vi "Create Output Channels.vi"(8 "error in (no error)":errorcluster, 11 "DAQmx Lockin Digitizer Driver in":refnum<class "DAQmx Synthesizer.lvclass">) -> (0 "error out":errorcluster, 3 "DAQmx Lockin Digitizer Driver out":refnum<class "DAQmx Synthesizer.lvclass">)   [LabVIEW 2021, in "DAQmx Synthesizer.lvclass"]
uses:
  DAQmx Synthesizer.lvclass
  C:/GitHub/NHMFL_Core/Libraries/Instruments/Pulse Driver/Lockin Digitizer Driver/Lockin Digitizer Driver.lvclass
  C:/GitHub/NHMFL_Core/Libraries/NI-DAQ/DAQmx Digitizer/DAQmx Digitizer.lvclass
  C:/GitHub/NHMFL_Core/Libraries/Instruments/Pulse Driver/Pulse Driver.lvclass
  DAQmx Digitizer/DAQmx Digitizer.lvclass/DAQmx Digitizer.ctl
  DAQmx Synthesizer.lvclass/DAQmx Synthesizer.ctl
  <vilib>/DAQmx/write.llb/DAQmx Write (Analog 1D Wfm NChan NSamp).vi
  DAQmx Digitizer/Read DAQmx Device Name.vi
  <vilib>/Waveform/WDTOps.llb/WDT Number of Waveform Samples DBL.vi
  <vilib>/DAQmx/create/channels.llb/DAQmx Create Channel (AO-Voltage-Basic).vi
  <vilib>/DAQmx/configure/timing.llb/DAQmx Timing (Sample Clock).vi
  <vilib>/DAQmx/configure/trigger.llb/DAQmx Start Trigger (Digital Edge).vi
  <vilib>/DAQmx/miscellaneous.llb/DAQmx Fill In Error Info.vi
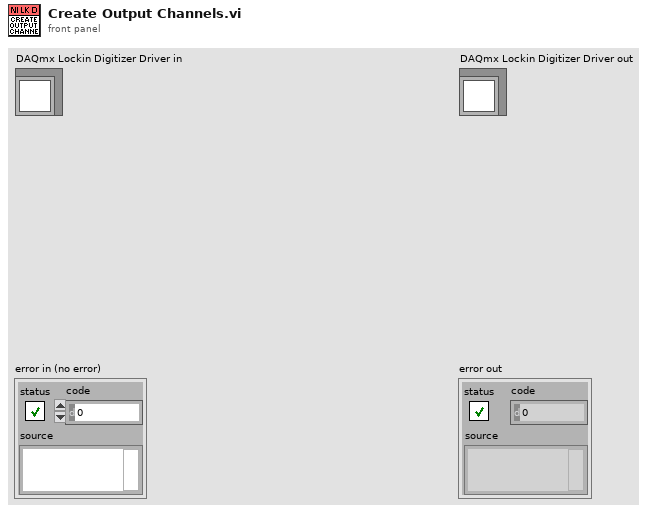
[diagram p1: front panel]
types:
  T1 = typedef "DAQmx Synthesizer Configuration.ctl" = cluster{"Channel names":string[], "Output channels":string, "Waveform file":path, "Offset":dbl, "Scale":dbl, "Ranges":dbl[], "Post-trigger delay":dbl, "Post-trigger duration":dbl, "Rate":dbl, "Re-name channels":string[], "Active channels":string, "External\nclock":bool}
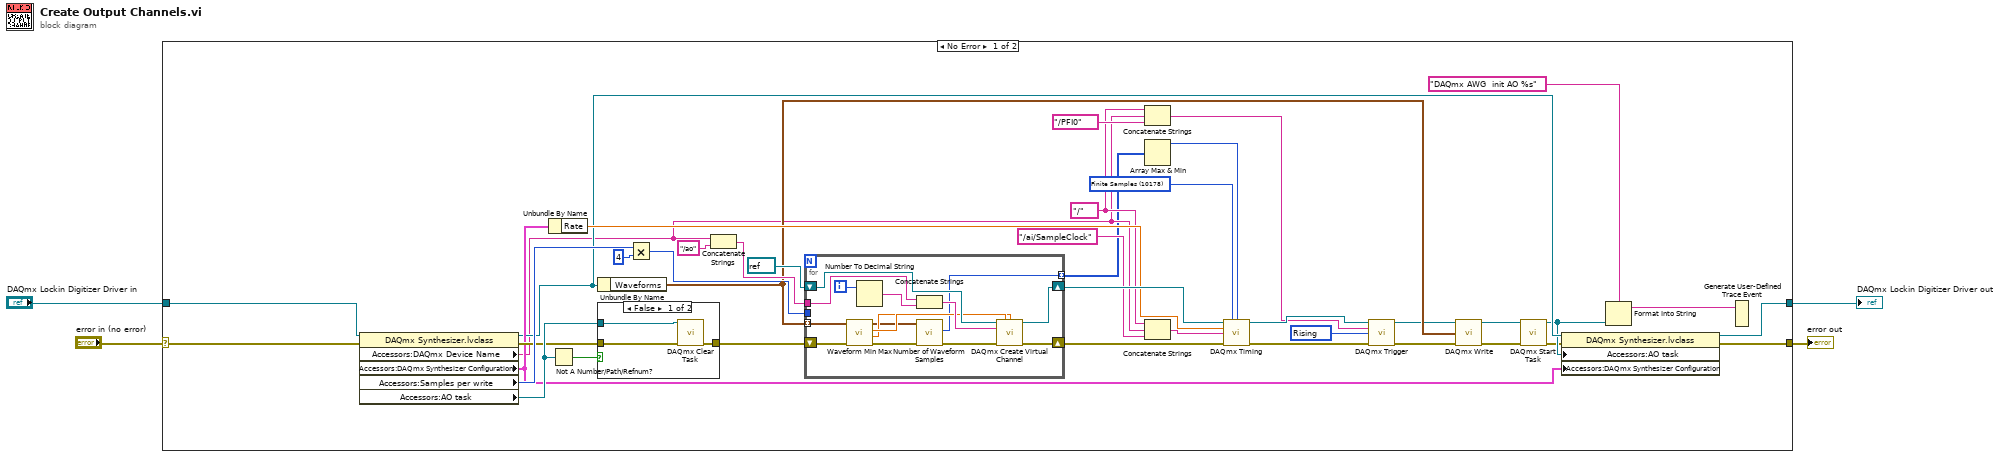
[diagram p0: block diagram]
diagram:
  n1 = case shown="No Error" "error in (no error)" {
    selector: "error in (no error)" -> [w41 w65]
    tunnel: [w43 w65] -> w3
    tunnel: [w44 w64] -> w1
    tunnel: "DAQmx Lockin Digitizer Driver in" -> [w42 w64]
    frame No Error {
      w15 = 10280 items=["Rising"=10280, "Falling"=10171] ("edge")
      w33 = 10178 items=["Finite Samples"=10178, "Continuous Samples"=10123, "Hardware Timed Single Point"=12522] ("sample mode")
      w13 = tag "/" ("string")
      n2 = property class="DAQmx Synthesizer.lvclass"(reference=w42, error in=w41) -> (reference out=w21:refnum<class "DAQmx Synthesizer.lvclass">, error out=w27:errorcluster, "Accessors:DAQmx Device Name"=w12:tag, "Accessors:DAQmx Synthesizer Configuration"=w22:T1, "Accessors:Samples per write"=w31:i32, "Accessors:AO task"=w28:refnum<k21>)
      n3 = Unbundle By Name(w22) -> ("Rate"=w23:dbl)
      n4 = Not A Number/Path/Refnum?(number/path/refnum=w28) -> (NaN/Path/Refnum?=w29:bool)
      n5 = Unbundle By Name(w21) -> ("Waveforms"=w18:waveform(dbl)[])
      n6 = case shown="False" w29 {
        tunnel: w28 -> [w47 _]
        tunnel: w27 -> [w46 w48]
        tunnel: [w45 w48] -> w26
        frame False {
          n7 = call <vilib>:"DAQmx Clear Task.vi"("task in"=w47, "error in"=w46) -> ("error out"=w45:errorcluster)  [unwired: 13 in]
        }
        frame True {
        }
      }
      n8 = Multiply(x=w31, y=4) -> (x*y=w30:i32)
      n9 = Concatenate Strings(w12, "/ao" ("string")) -> (w38:string)
      n10 = for {
        shift-right: [w62] -> w37
        shift-left: w26 -> [w53]
        shift-right: [w63] -> w36
        shift-left: refnum<k21> refnum ("task out") -> [w61]
        tunnel: w38 -> [w58]
        tunnel: w30 -> [_]
        tunnel: w18 -> [w56] mode=indexing
        tunnel: [w51] -> w6 mode=indexing
        i -> [w59]
        n11 = call <vilib>:"Waveform Min Max.vi"("error in (no error)"=w53, "waveform in"=w56) -> ("error out"=w50:errorcluster, "Y min"=w54:dbl, "Y max"=w55:dbl, "waveform out"=w52:waveform(dbl))  [unwired: 4 in, 2 out]
        n12 = Number To Decimal String(number=w59) -> (decimal integer string=w60:string)  [unwired: 1 in]
        n13 = Concatenate Strings(w58, w60) -> (w57:string)
        n14 = call-poly <vilib>:"Number of Waveform Samples.vi"("error in (no error)"=w50, "waveform in"=w52) -> ("error out"=w49:errorcluster, "number of samples"=w51:i32)  [unwired: 7 in, 1 out]
        n15 = call-poly <vilib>:"DAQmx Create Virtual Channel.vi"("task in"=w61, "maximum value"=w55, "minimum value"=w54, "physical channels"=w57, "error in"=w49) -> ("task out"=w63:refnum<k21>, "error out"=w62:errorcluster)  [unwired: 9 in]
      }
      n16 = Concatenate Strings(w13, w12, tag "/PFI0" ("string")) -> (w11:string)
      n17 = Array Max & Min(array=w6) -> (max value=w5:i32)  [unwired: 3 out]
      n18 = Concatenate Strings(w13, w12, "/ai/SampleClock" ("string")) -> (w34:string)
      n19 = call-poly <vilib>:"DAQmx Timing.vi"("task/channels in"=w36, "sample mode"=w33, "samples per channel"=w5, "rate"=w23, "source"=w34, "error in"=w37) -> ("task out"=w17:refnum<k21>, "error out"=w20:errorcluster)  [unwired: 8 in]
      n20 = call-poly <vilib>:"DAQmx Trigger.vi"("task/channels in"=w17, "source"=w11, "edge"=w15, "error in"=w20) -> ("task out"=w16:refnum<k21>, "error out"=w19:errorcluster)  [unwired: 10 out]
      n21 = call-poly <vilib>:"DAQmx Write.vi"("task/channels in"=w16, "data"=w18, "error in"=w19) -> ("task out"=w10:refnum<k21>, "error out"=w7:errorcluster)  [unwired: 10 in, 1 out]
      n22 = call <vilib>:"DAQmx Start Task.vi"("task/channels in"=w10, "error in"=w7) -> ("task out"=w9:refnum<k21>, "error out"=w8:errorcluster)  [unwired: 12 out]
      n23 = property class="DAQmx Synthesizer.lvclass"(reference=w21, error in=w8, "Accessors:AO task"=w9, "Accessors:DAQmx Synthesizer Configuration"=w22) -> (reference out=w44:refnum<class "DAQmx Synthesizer.lvclass">, error out=w43:errorcluster)
      n24 = Format Into String(format string="DAQmx AWG  init AO %s" ("string"), w9) -> (resulting string=w24:string)  [unwired: 2 in, 1 out]
      n25 = Generate User-Defined Trace Event(2:w24) -> ()  [unwired: 1 in]
    }
    frame Error {
    }
  }
  "error out" <- w3
  "DAQmx Lockin Digitizer Driver out" <- w1
